vi "Handle Error.vi"(8 "error in (no error)":errorcluster, 11 "AMS Gas in":refnum<class "AMS Gas.lvclass">) -> (0 "error out":errorcluster, 2 "stop actor?":bool=TRUE, 3 "AMS Gas out":refnum<class "AMS Gas.lvclass">)   [LabVIEW 2015, in "AMS UI.lvlib" / "AMS Gas.lvclass"]
doc: "(<B>Filename</B>: Actor Framework.lvlib:Actor.lvclass:Handle Error.vi)\n\nDefines how the actor handles an error that occurred while processing a message.\n\nBy default, this method does nothing except stop the actor. This method also treats error code 43 (coming from <B>error in</B>) as a sign that the actor shut down normally. In this situation, the Handle Error method does not return the error on <B>error out</B>, meaning the actor's caller will not receive it. All other error codes will be returned on <B>error out</B>.\n\nA descendant class may override this method to change this behavior."
uses:
  AMS Gas.lvclass
  <vilib>/Utility/error.llb/DialogType.ctl
  <vilib>/ActorFramework/Actor/Actor.lvclass
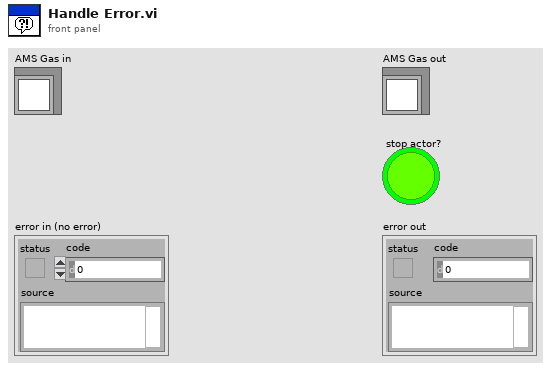
[diagram p1: front panel]
types:
  T1 = typedef "DialogType.ctl" = u16
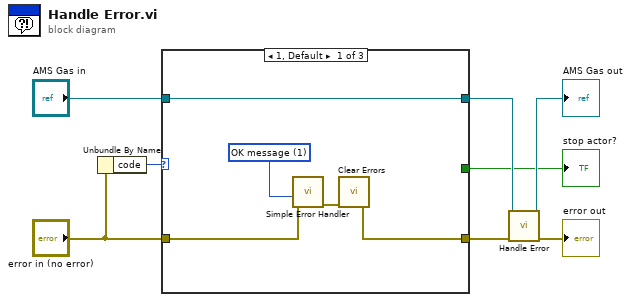
[diagram p0: block diagram]
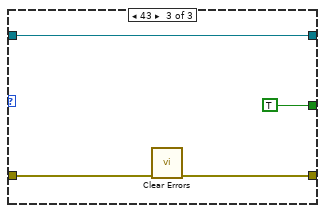
[diagram p3: hidden frame]
diagram:
  n1 = Unbundle By Name("error in (no error)") -> ("code"=w6:i32)
  n2 = case shown="1, Default" w6 {
    tunnel: "error in (no error)" -> [w12 w15 w17]
    tunnel: [w9 w15 w16] -> w4
    tunnel: "AMS Gas in" -> [w13 w14 w19]
    tunnel: [w13 w14 w19] -> w2
    tunnel: [_ _ TRUE ("stop actor?")] -> w1
    frame 1, Default {
      w11 = T1 1 items=["no dialog", "OK message", "continue or stop message", "OK message + warnings", "continue/stop + warnings"] ("type of dialog (OK msg:1)")
      n3 = call <vilib>:"Simple Error Handler.vi"("type of dialog (OK msg:1)"=w11, "error in (no error)"=w12) -> ("error out"=w10:errorcluster)  [unwired: 3 in, 4 out]
      n4 = call <vilib>:"Clear Errors.vi"("error in (no error)"=w10) -> ("error out"=w9:errorcluster)  [unwired: 5 in, 1 out]
    }
    frame 0 {
    }
    frame 43 {
      n5 = call <vilib>:"Clear Errors.vi"("error in (no error)"=w17) -> ("error out"=w16:errorcluster)  [unwired: 5 in, 1 out]
    }
  }
  "stop actor?" <- w1
  n6 = call-parent "Handle Error.vi"("error in (no error)"=w4, "Actor in"=w2) -> ("error out"=→"error out":errorcluster, "Actor out"=→"AMS Gas out":refnum<class "AMS Gas.lvclass">)  [unwired: 7 in, 1 out]
